vi "setPinvA.vi"(8 "error in (no error)":errorcluster, 10 "Truncation Threshold":dbl=0.0001, 11 "OptStateEsti in":refnum<class "OptStateEsti.lvclass">) -> (0 "error out":errorcluster, 3 "OptStateEsti out":refnum<class "OptStateEsti.lvclass">)   [LabVIEW 2016, in "OfcFunc.lvlib" / "OptStateEsti.lvclass"]
doc: "Set the pueudo-inversed matrix A with the truncation."
uses:
  OptStateEsti.lvclass
  OptStateEsti.lvclass/OptStateEsti.ctl
  <vilib>/Analysis/_algsub.llb/Real PseudoInverse Matrix.vi
  <vilib>/Analysis/Matrix/Numeric/Conversions/Array To Matrix - RA2.vi
  <vilib>/Analysis/Matrix/Numeric/Conversions/Matrix To Array - RM.vi
  <vilib>/Analysis/NI_AALPro.lvlib
  <vilib>/Analysis/Matrix/NI_Matrix.lvlib
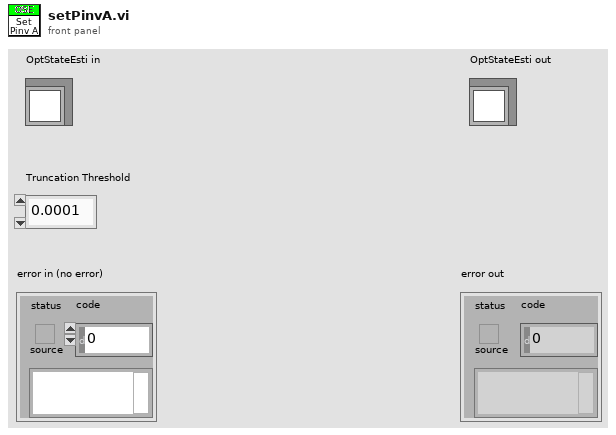
[diagram p1: front panel]
types:
  T1 = typedef "NI_Matrix.lvlib/RealMatrix.ctl" = dbl[][]
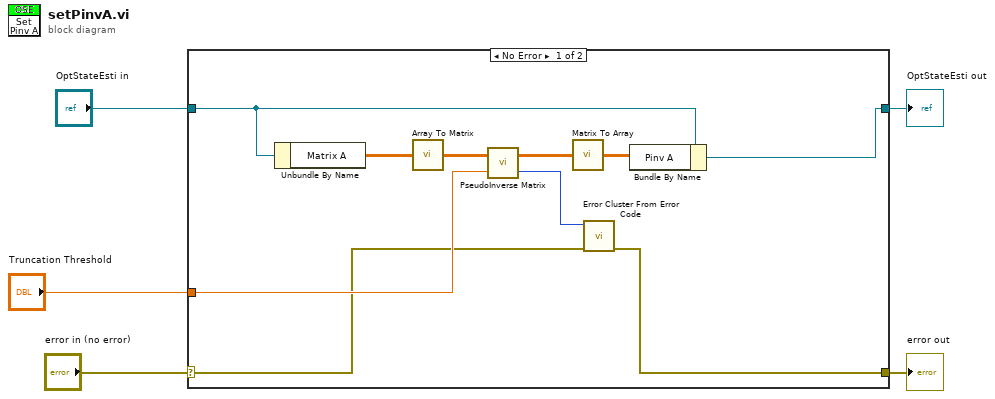
[diagram p0: block diagram]
diagram:
  n1 = case shown="No Error" "error in (no error)" {
    selector: "error in (no error)" -> [w8 w17]
    tunnel: [w10 w17] -> w4
    tunnel: [w15 w16] -> w2
    tunnel: "OptStateEsti in" -> [w7 w16]
    tunnel: "Truncation Threshold" -> [w12 _]
    frame No Error {
      n2 = Unbundle By Name(w7) -> ("Matrix A"=w6:dbl[][])
      n3 = call-poly <vilib>:"Array To Matrix.vi"("Real 2D Array"=w6) -> ("Real Matrix"=w9:T1)
      n4 = call-poly <vilib>:"PseudoInverse Matrix.vi"("tolerance"=w12, "Input Matrix"=w9) -> ("error"=w11:i32, "PseudoInverse Matrix"=w13:T1)
      n5 = call-poly <vilib>:"Matrix To Array.vi"("Real Matrix"=w13) -> ("Real 2D Array"=w14:dbl[][])
      n6 = call <vilib>:"Error Cluster From Error Code.vi"("error in (no error)"=w8, "error code (0)"=w11) -> ("error out"=w10:errorcluster)  [unwired: 7 in]
      n7 = Bundle By Name(cluster=w7, "Pinv A"=w14) -> (w15:refnum<class "OptStateEsti.lvclass">)
    }
    frame Error {
    }
  }
  "error out" <- w4
  "OptStateEsti out" <- w2
